vi "Set View Date.vi"(8 "error in (no error)":errorcluster, 10 "Date":string, 11 "Tree in":refnum<class "Tree.lvclass">) -> (0 "error out":errorcluster, 3 "Tree out":refnum<class "Tree.lvclass">)   [LabVIEW 2015, in "MDSplus.lvlib" / "Tree.lvclass"]
doc: "Set the version date: all read data will refer to the version active to that date."
uses:
  Tree.lvclass
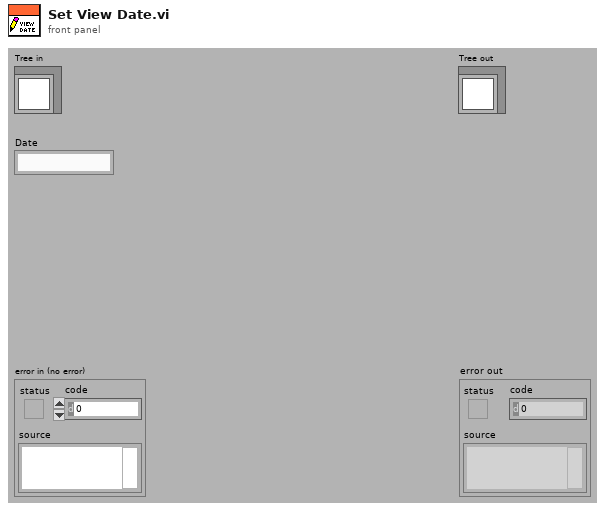
[diagram p1: front panel]
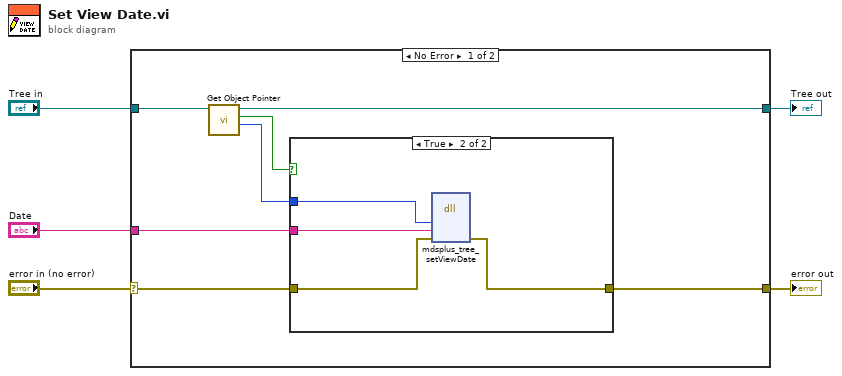
[diagram p0: block diagram]
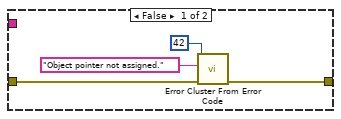
[diagram p2: hidden frame]
diagram:
  n1 = case shown="No Error" "error in (no error)" {
    selector: "error in (no error)" -> [w8 w22]
    tunnel: [w7 w22] -> w4
    tunnel: [w11 w21] -> w2
    tunnel: "Tree in" -> [w12 w21]
    tunnel: "Date" -> [w6 _]
    frame No Error {
      n2 = call-dynamic "Get Object Pointer.vi"("Tree in"=w12) -> ("Object Pointer"=w9:i64, "Assigned object pointer?"=w10:bool, "Tree out"=w11:refnum<class "Tree.lvclass">)  [unwired: 8 in]
      n3 = case shown="True" w10 {
        tunnel: w9 -> [_ w20]
        tunnel: w8 -> [w14 w19]
        tunnel: [w13 w18] -> w7
        tunnel: w6 -> [_ w17]
        frame False {
          n4 = call <vilib>:"Error Cluster From Error Code.vi"("error in (no error)"=w14, "error message (\"\")"="Object pointer not assigned." ("error message (\"\")"), "error code (0)"=42) -> ("error out"=w13:errorcluster)  [unwired: 6 in]
        }
        frame True {
          n5 = dll-call lib="MDSobjectsLVShr" fn="mdsplus_tree_setViewDate"("lvTreePtr"=w20, "dateIn"=w17, "error"=w19) -> ("error"=w18:errorcluster)  [unwired: 6 in, 2 out]
        }
      }
    }
    frame Error {
    }
  }
  "error out" <- w4
  "Tree out" <- w2
